vi "JSON to LVObject - Warning Input - Returns Same Warning.vi"() -> ()   [LabVIEW 2017, in "JSON Serializable Serializer Tests.lvlib"]
uses:
  JSON Serializable Serializer Tests.lvlib
  JSON Serializable Serializer/JSON Serializable Serializer.lvclass
  <vilib>/Utility/error.llb/Error Cluster From Error Code.vi
  <vilib>/addons/_JKI Toolkits/Caraya/classes/Assert/Assert Equal Value_Variant.vi
  <vilib>/ErrorRing/Error Ring.xnode
  <vilib>/addons/_JKI Toolkits/Caraya/classes/Test/Test.lvclass
  <vilib>/addons/_JKI Toolkits/Caraya/classes/Assert/Assert.lvclass
panel:
  out "error out":errorcluster
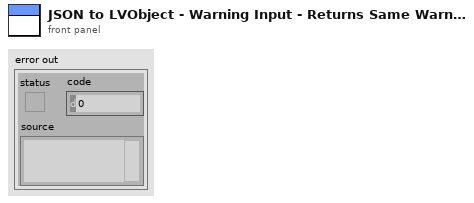
[diagram p1: front panel]
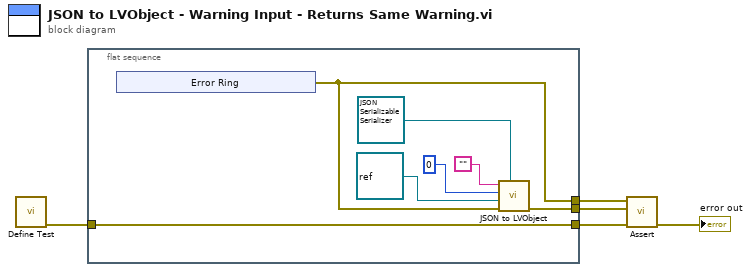
[diagram p0: block diagram]
diagram:
  n1 = call <vilib>:"Define Test.vi"() -> ("error out"=w2:errorcluster)  [unwired: 11 in]
  n2 = flat-sequence {
    tunnel: [w12] -> w5
    tunnel: [w11] -> w4
    tunnel: [w10] -> w3
    tunnel: w2 -> [w10]
    frame #0 {
      n3 = xnode "Error Ring"() -> ("error out"=w11:errorcluster)
      n4 = call-dynamic "JSON to LVObject.vi"("JSON Serializer in"=refnum<class "JSON Serializable Serializer.lvclass"> refnum ("JSON Serializer.lvclass"), "error in (no error)"=w11, "Object Type"=refnum<class> refnum ("Type"), "Offset"=0, "JSON"="") -> ("error out"=w12:errorcluster)  [unwired: 5 in, 1 out]
    }
  }
  n5 = call-poly <vilib>:"Assert.vi"("error in (no error)"=w3, "Y"=w5, "X"=w4) -> ("error out"=→"error out":errorcluster)  [unwired: 8 in]
